vi "AuMT8852B Identification Query.vi"(8 "error in (no error)":errorcluster, 11 "VISA session":refnum<visa-resource-name>) -> (0 "error out":errorcluster, 2 "error code":i32, 3 "VISA session out":refnum<visa-resource-name>, 4 "Identification":string="ANRITSU,MT8850A,0,0")   [LabVIEW 2017]
doc: "Anritsu MT8852B Bluetooth Tester\n\nOUTPUTS\nIdentification - the manufacturer, model, serial number, and firmware version of the instrument."
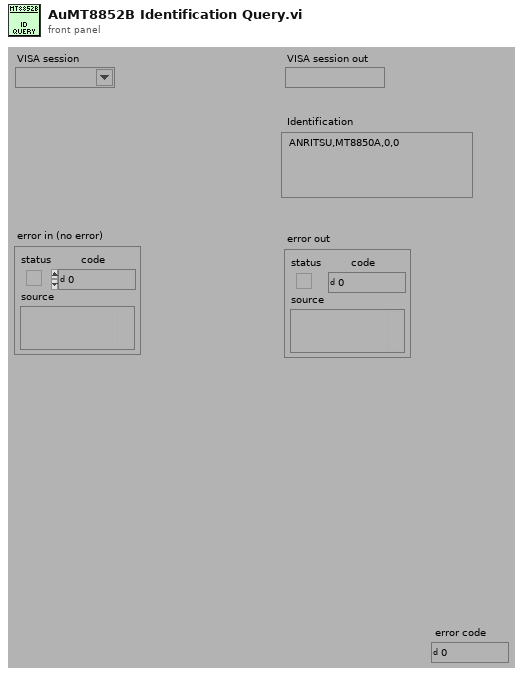
[diagram p1: front panel]
types:
  T1 = enum16{"Simulate", "Range check", "Cache", "Query instrument status"}
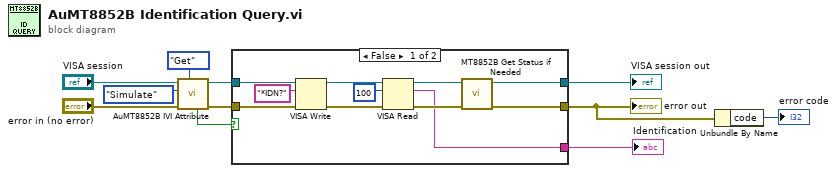
[diagram p0: block diagram]
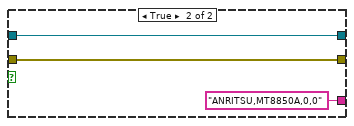
[diagram p2: hidden frame]
diagram:
  n1 = call <instrlib>:"AuMT8852B IVI Attribute.vi"("Set/Get (Set)"=enum16{"Set", "Get"}."Get", "error in (no error)"="error in (no error)", "Flag (Simulate)"=T1."Simulate", "VISA session"="VISA session") -> ("error out"=w8:errorcluster, "VISA session out"=w10:refnum<visa-resource-name>, "Value out"=w4:bool)  [unwired: 5 in]
  n2 = case shown="False" w4 {
    tunnel: [w17 w25] -> w11
    tunnel: [w16 w24] -> w1
    tunnel: w10 -> [w21 w25]
    tunnel: w8 -> [w20 w24]
    tunnel: [w12 "ANRITSU,MT8850A,0,0" ("read buffer")] -> w3
    frame False {
      n3 = VISA Write(VISA resource name=w21, write buffer="*IDN?" ("write buffer (\"\")"), error in (no error)=w20) -> (VISA resource name out=w14:refnum<visa-resource-name>, error out=w15:errorcluster)  [unwired: 1 out]
      n4 = VISA Read(VISA resource name=w14, byte count=u32 100 ("byte count (0)"), error in (no error)=w15) -> (VISA resource name out=w19:refnum<visa-resource-name>, read buffer=w12:string, error out=w18:errorcluster)  [unwired: 1 out]
      n5 = call <instrlib>:"MT8852B Get Status if Needed.vi"("error in (no error)"=w18, "VISA session"=w19) -> ("error out"=w16:errorcluster, "VISA session out"=w17:refnum<visa-resource-name>)  [unwired: 8 in]
    }
    frame True {
      (unwired) "" ("Response")
    }
  }
  "error out" <- w1
  "VISA session out" <- w11
  "Identification" <- w3
  n6 = Unbundle By Name(w1) -> ("code"=→"error code":i32)
